vi "Renishaw-XL80_GetSignalStrength.vi"(8 "error in (no error)":errorcluster, 11 "Renishaw-XL80 in":refnum<class "Renishaw-XL80.lvclass">) -> (0 "error out":errorcluster, 2 "Signal Strength":i16, 3 "Renishaw-XL80 out":refnum<class "Renishaw-XL80.lvclass">)   [LabVIEW 2024, in "Renishaw-XL80.lvclass"]
doc: "This read only property returns the current signal strength of the ML10.\n\nDefinition\nHRESULTget_SignalStrength( [out, retval] short* pVal);\nParameters\npVal\nA variable that will be set to the signal strength of the ML10.\n\nComments\nThis property will return with an HRESULT of E_FAIL if the client has not previously connected to a DX10 by calling Connect.\n\nOtherwise the property will normally return an HRESULT of S_OK. However, it will return E_POINTER if the client supplies a null pointer for pVal.\n\nIf the ML10 is not responding then the signal strength will return the last known good value.\n\nThe signal strength is a value between 0 and 31, where 31 implies 100% signal strength. Note that it is customary to truncate any signal strength display meter at 26. So the user doesn't waste time trying to achieve signal strengths close to 100% which will have no benefit to measurement accuracy."
uses:
  Renishaw-XL80.lvclass
  Renishaw-XL80.lvclass/Renishaw-XL80.ctl
  D:/A.C.M/Example CSharp_64/bin/Debug/Interop.DX10SDKADAPTORLib.dll
  Example CSharp_64/bin/Debug/Interop.DX10SDKADAPTORLib.dll
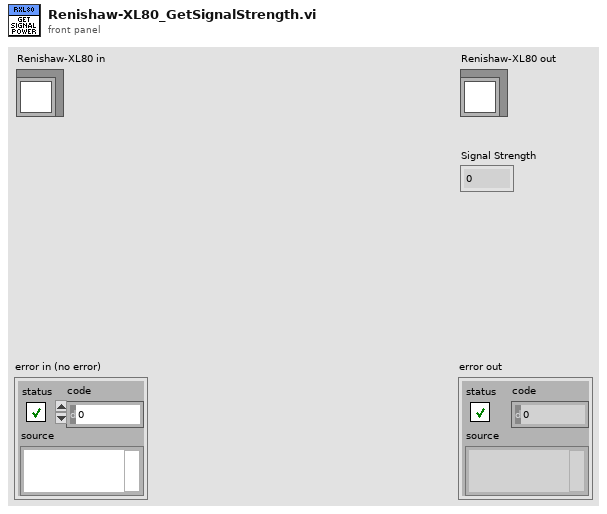
[diagram p1: front panel]
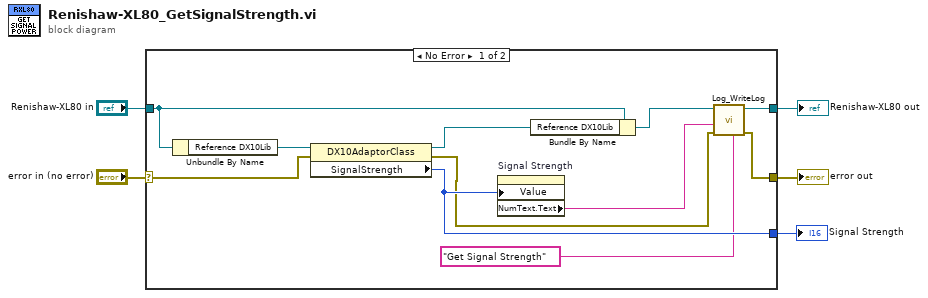
[diagram p0: block diagram]
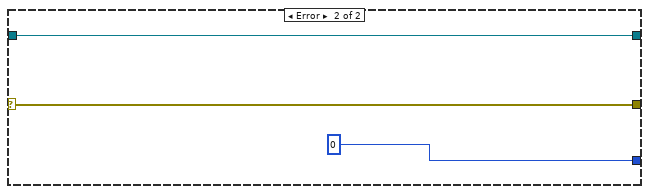
[diagram p2: hidden frame]
diagram:
  n1 = case shown="No Error" "error in (no error)" {
    selector: "error in (no error)" -> [w15 w19]
    tunnel: [w7 w19] -> w4
    tunnel: [w11 w18] -> w2
    tunnel: "Renishaw-XL80 in" -> [w14 w18]
    tunnel: [w10 i16 0 ("SignalStrength")] -> w1
    frame No Error {
      n2 = Unbundle By Name(w14) -> ("Reference DX10Lib"=w16:refnum<k24>)
      n3 = property class="DX10AdaptorClass"(reference=w16, error in=w15) -> (reference out=w13:refnum<k24>, error out=w6:errorcluster, "SignalStrength"=w10:i16)
      n4 = property on="Signal Strength" class="DigNum (strict)"("Value"=w10) -> ("NumText.Text"=w9:string)  [unwired: 2 in, 2 out]
      n5 = Bundle By Name(cluster=w14, "Reference DX10Lib"=w13) -> (w12:refnum<class "Renishaw-XL80.lvclass">)
      n6 = call-dynamic "Log_WriteLog.vi"("Additional text"="Get Signal Strength", "error in (no error)"=w6, "Response"=w9, "Log in"=w12) -> ("error out"=w7:errorcluster, "Log out"=w11:refnum<class "Renishaw-XL80.lvclass">)  [unwired: 6 in]
    }
    frame Error {
    }
  }
  "error out" <- w4
  "Renishaw-XL80 out" <- w2
  "Signal Strength" <- w1
